vi "TestHB_Emb_1_arraysender.vi"() -> ()   [LabVIEW 2012]
doc: "SciScan 1.2 160622"
uses:
  SubVIs/Master Slave messaging Flags.ctl
  Custom Controls and Typedefs/HB_Error Conditions Cluster.ctl
  Custom Controls and Typedefs/Heartbeat information cluster.ctl
  Custom Controls and Typedefs/Heartbeat Event Source.ctl
  Custom Controls/Heartbeat_States.ctl
  SubVIs/Heartbeat state manager Input VI names.ctl
  Custom Controls and Typedefs/HB Actionable Event.ctl
  Custom Controls and Typedefs/HFG Commands.ctl
panel:
  in  "Cancel Sending":bool
  in  "Send command":bool
  out "Master instr received":i32
  out "Slave conf received":i32
  out "Heartbeat information cluster":T1
  out "Error conditions Cluster":T4
  out "Master-Slave messaging Flags":T5={"Instruction available"=TRUE, "Slave action completed"=TRUE, "Slave Ready?"=FALSE}
  in  "stop":bool
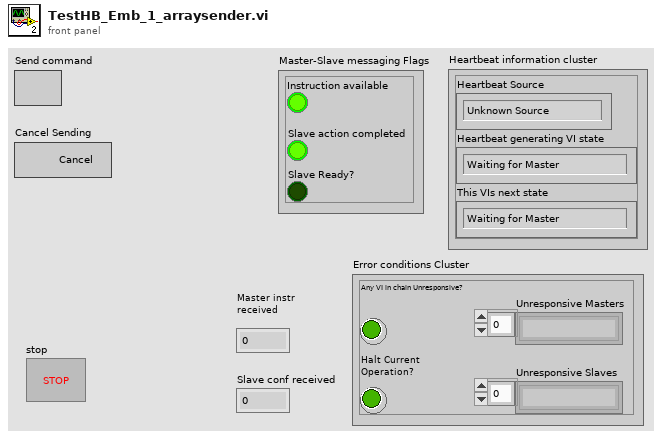
[diagram p1: front panel]
types:
  T1 = typedef "Heartbeat information cluster.ctl" = cluster{"Heartbeat Source":T2, "Heartbeat generating VI state":T3, "This VIs next state":T3}
  T2 = typedef "Heartbeat Event Source.ctl" = enum16{"Unknown Source", "Timeout", "This VI", "Master", "Slave"}
  T3 = typedef "Heartbeat_States.ctl" = enum16{"Waiting for Master", "Instruction Issued", "Waiting for Slave Completion", "Completed", "Cancelled", "Failed", "Broken Link"}
  T4 = typedef "HB_Error Conditions Cluster.ctl" = cluster{"Any VI in chain Unresponsive?":bool, "Halt Current Operation?":bool, "Unresponsive Masters":string[], "Unresponsive Slaves":string[]}
  T5 = typedef "Master Slave messaging Flags.ctl" = cluster{"Instruction available":bool, "Slave action completed":bool, "Slave Ready?":bool}
  T6 = enum8{"Enabled", "Disabled", "Disabled and Grayed Out"}
  T7 = typedef "HB Actionable Event.ctl" = enum16{"Master instruction event", "Slave ready event", "Slave unavailable event", "Cancelled or Failed event", "Slave action complete event", "QUIT", "Broken Link", "Recovered from Broken Link"}
  T8 = typedef "Heartbeat state manager Input VI names.ctl" = cluster{"Current VI name":string, "Master VI Names":string[], "Slave VI Names":string[]}
  T9 = typedef "HFG Commands.ctl" = enum16{"Set", "Get", "Initialize"}
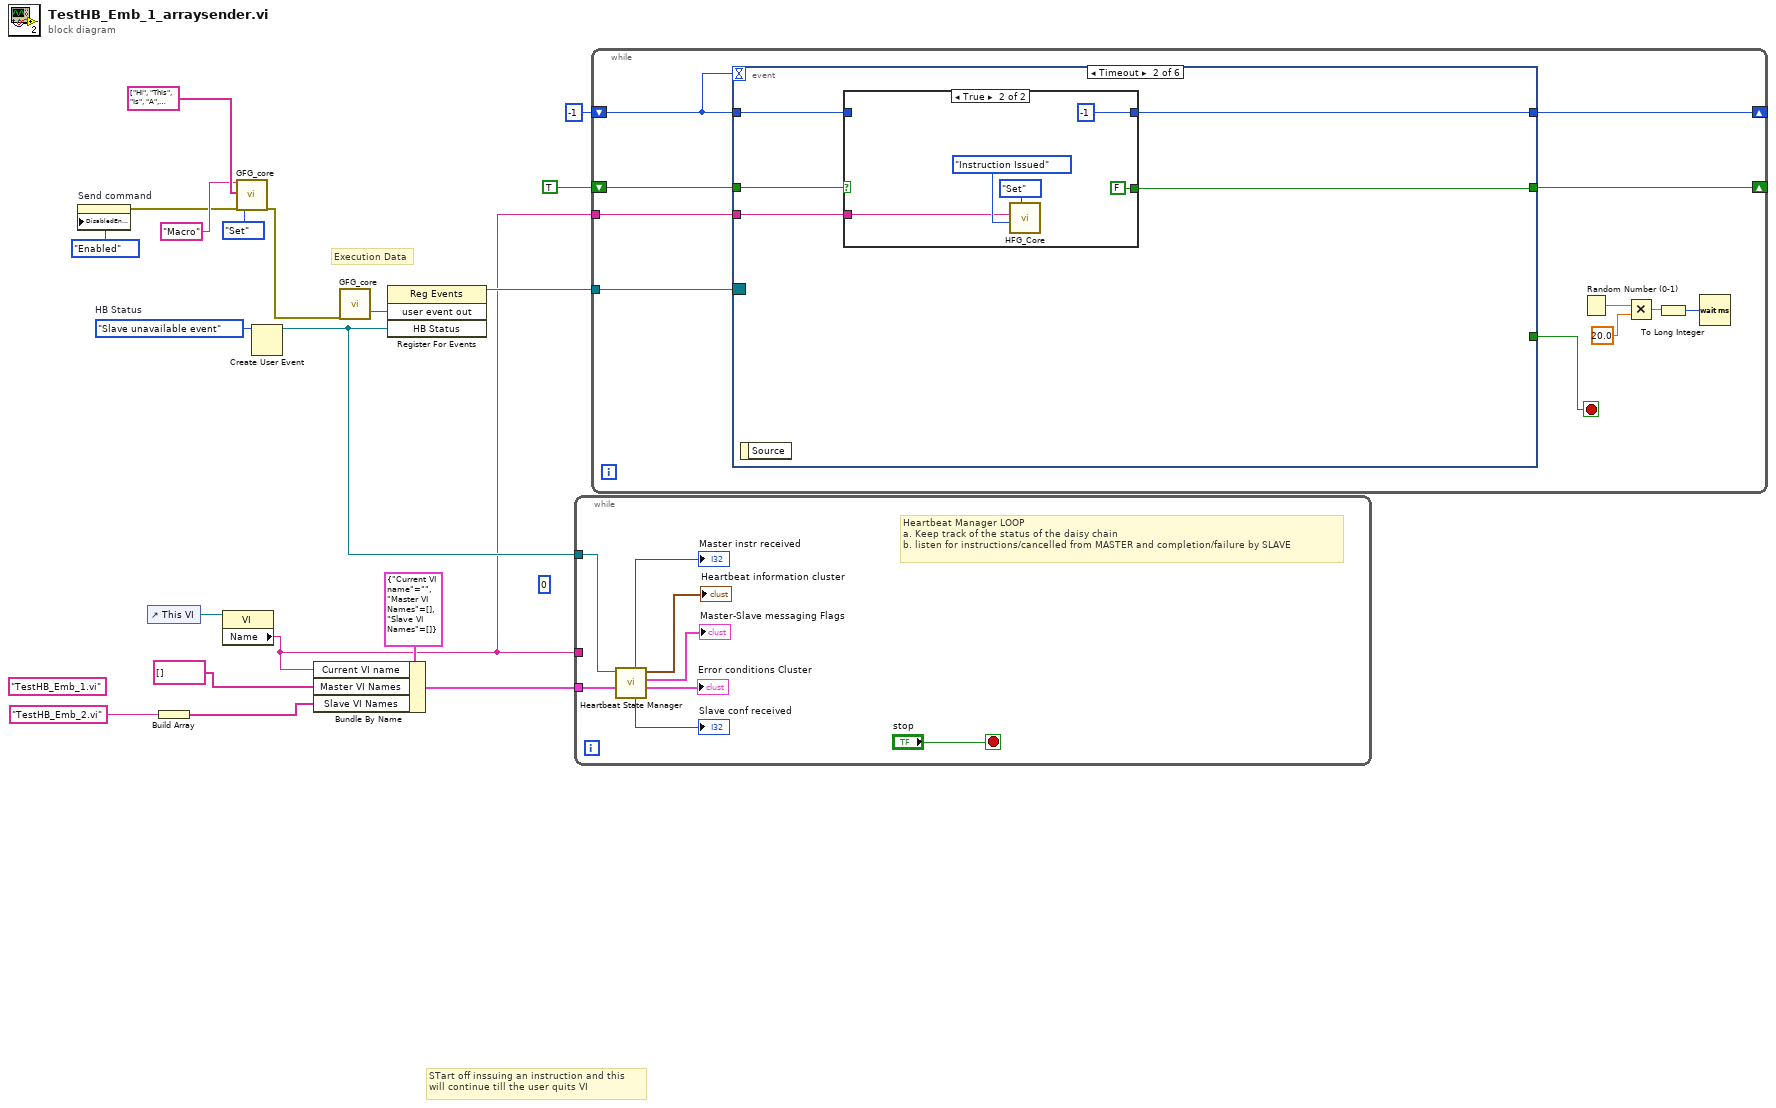
[diagram p0: block diagram]
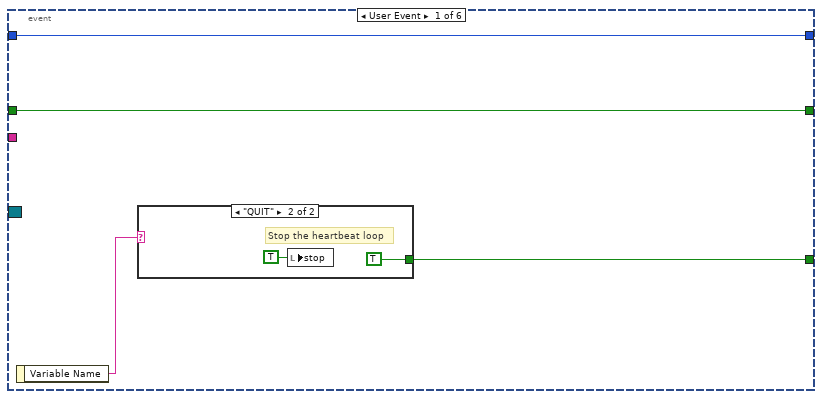
[diagram p2: hidden frame]
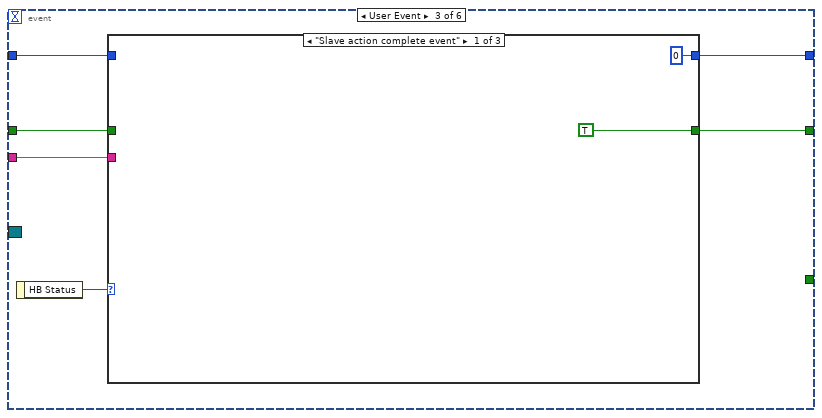
[diagram p5: hidden frame]
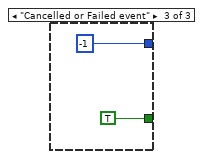
[diagram p7: hidden frame]
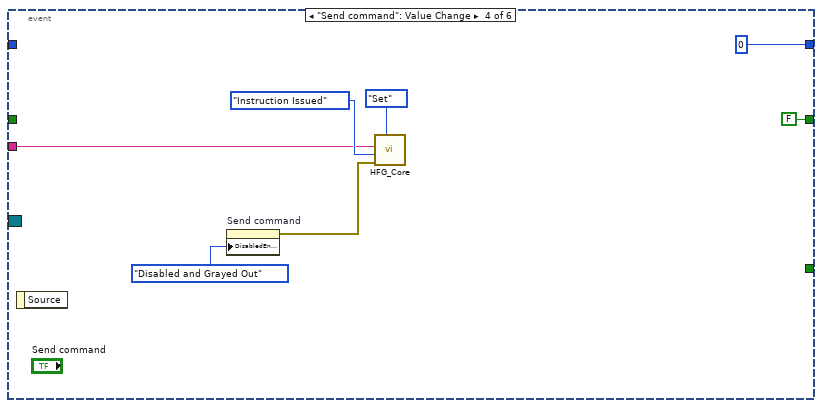
[diagram p8: hidden frame]
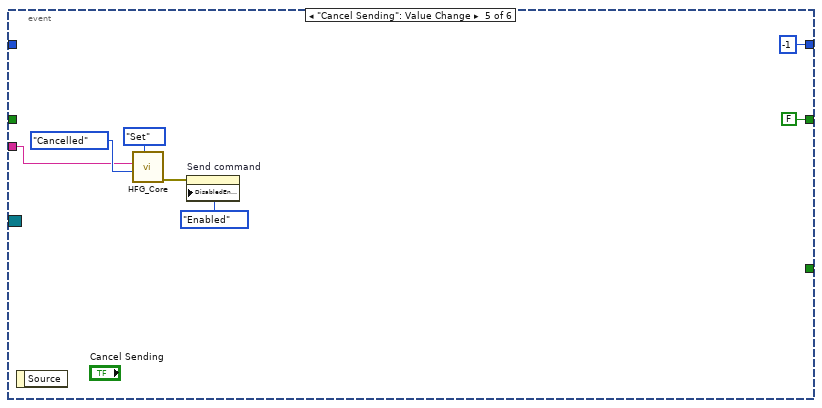
[diagram p9: hidden frame]
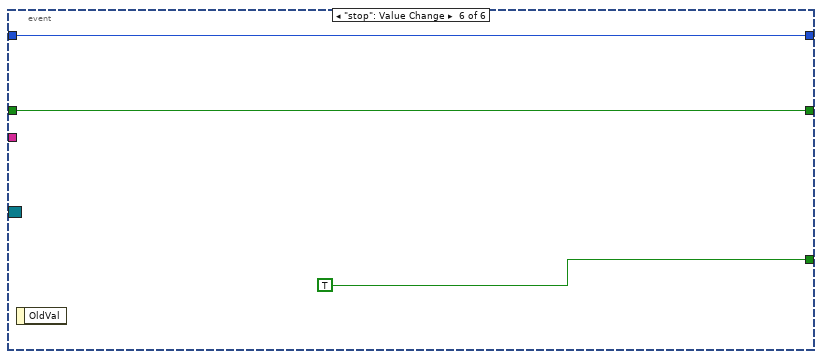
[diagram p10: hidden frame]
diagram:
  w12 = HB_Actionable_Event."Slave unavailable event"  # HB Status
  (unwired) 0
  (unwired) "TestHB_Emb_1.vi"
  # "STart off inssuing an instruction and this \nwill continue till the user quits VI"
  # "Execution Data"
  n1 = property on="Send command" class="Bool"("DisabledEnum"=T6."Enabled" ("Disabled")) -> (error out=w2:errorcluster)  [unwired: 2 in, 1 out]
  n2 = control-ref of="This VI"() -> (w17:refnum<vi>)
  n3 = Build Array("TestHB_Emb_2.vi") -> (w15:string[])
  n4 = property class="VI"(reference=w17) -> ("Name"=w9:string)  [unwired: 1 in, 2 out]
  n5 = call "GFG_core.vi"("Variable Name in"="Macro", "Variant in"=string[] ["Hi", "This", "Is", "A", "Test", "fg", "fgg", "ghg", "gh", "gh", "gh", "h", "hg", "f", "gn", "dghs", "dgh", "dghd", "dh", "d", "dghz", "afd", "gh", "afdg", "adfg", "dafg", "dfgh", "adfg", "dfg", "fdg", "dafg", "a", "hz", "fg", "dafg", "fdg", "adfg", "ag", "hadfg", "dfg", "adfg", "afg", "gjsgh", "dfhg", "dfg", "dfg", "jadfgh", "fhad", "hdgfh", "adfg", "hsdhgf", "adfg", "hdgfh", "fgg", "hdafh", "fdghfd", "hgsdha", "adfga", "ghadfh", "fdh", "fhjda", "fgasd", "hdha", "ahfdjhs", "dha", "hjg", "jgfsj", "adgh", "sdgh", "dsgjs", "adfh", "sdgha", "fdha", "dfhhs", "hgshjs", "gjhs", "gdh", "sgfh", "sgh", "gjhs", "hfdj", "dsfhj", "dfh", "jdhj", "fhjd", "ghfg", "fhjd", "dfjdf", "hjdf", "gjdfgj", "fhjd", "jkkg", "kfdh", "dfhjsd", "fhj", "fhj", "sfgj", "sfgjsf", "fgjgfj", "sfgjsf", "jfghjsgf", "fghjsf", "fsghj"] ("Array"), "error in (no error)"=w2, "Action"=enum16{"Init", "Set", "Get", "Clear"}."Set") -> ("error out"=w4:errorcluster)  [unwired: 9 in, 6 out]
  n6 = Create User Event(user event datatype=w12) -> (user event=w11:refnum<user-event>)  [unwired: 1 in, 1 out]
  n7 = Bundle By Name(cluster=T8 {"Current VI name"="", "Master VI Names"=[], "Slave VI Names"=[]} ("Heartbeat state manager Input VI names 2"), "Current VI name"=w9, "Master VI Names"=string[] [], "Slave VI Names"=w15) -> (w16:T8)
  n8 = call "GFG_core.vi"("error in (no error)"=w4) -> ("user event out"=w14:refnum<user-event>)  [unwired: 12 in, 6 out]
  n9 = register-events(w14, w11) -> (reference out=w13:refnum<event-registration>)  [unwired: 2 in, 1 out]
  n10 = while {
    tunnel: w16 -> [w27]
    tunnel: w9 -> [_]
    tunnel: w11 -> [w21]
    stop <- "stop" stop-if-true
    # "Heartbeat Manager LOOP \na. Keep track of the status of the daisy chain\nb. listen for instructions/cancelled from MASTER and completion/failure by SLAVE"
    n11 = call "Heartbeat State Manager.vi"("Heartbeat state manager Input VI names"=w27, "HB Command Event IN"=w21) -> ("Error conditions Cluster"=→"Error conditions Cluster":T4, "Master-Slave messaging Flags"=→"Master-Slave messaging Flags":T5, "Heartbeat information cluster"=→"Heartbeat information cluster":T1, "Slave Completions Received"=→"Slave conf received":i32, "Master Instructions Issued"=→"Master instr received":i32)  [unwired: 4 in, 1 out]
  }
  n12 = while {
    tunnel: w13 -> [w38]
    tunnel: w9 -> [w36]
    shift-right: [w34] -> _
    shift-left: TRUE ("slave ready") -> [w35]
    shift-right: [w29] -> _
    shift-left: -1 -> [w28]
    stop <- w37 stop-if-true
    n13 = event shown="[1] Timeout" {
      selector: w38 -> [_ _ _ _ _ _]
      dyn-events: _ -> [_ _ _ _ _ _]
      timeout: w28 -> [_ _ _ _ _ _]
      tunnel: [w41 _ _ _ _ TRUE] -> w37
      tunnel: w36 -> [_ w48 w61 w73 w80 _]
      tunnel: w35 -> [w40 w49 w60 _ _ w84]
      tunnel: [w40 w46 w59 FALSE ("slave ready") FALSE ("slave ready") w84] -> w34
      tunnel: [w39 w45 w57 0 -1 w83] -> w29
      tunnel: w28 -> [w39 w47 w58 _ _ w83]
      event User Event {
        n14 = event-data() -> ("Variable Name"=w42:string)  [unwired: 1 in]
        n15 = case shown="\"QUIT\"" w42 {
          tunnel: [_ TRUE] -> w41
          frame "False", Default {
          }
          frame "QUIT" {
            # "Stop the heartbeat loop"
            n16 = local write "stop"(TRUE ("stop")) -> ()
          }
        }
      }
      event Timeout {
        n17 = event-data() -> ()  [unwired: 1 in, 1 out]
        n18 = case shown="True" w49 {
          selector: w49 -> [w51 _]
          tunnel: w48 -> [_ w54]
          tunnel: w47 -> [w50 _]
          tunnel: [w51 FALSE] -> w46
          tunnel: [w50 -1] -> w45
          frame False {
          }
          frame True {
            n19 = call "HFG_Core.vi"("HFG Commands"=HFG_Commands."Set", "Heartbeat state IN"=Heartbeat_States."Instruction Issued", "VI Name (Calling VIs name by default)"=w54) -> ()  [unwired: 5 in, 4 out]
          }
        }
      }
      event User Event {
        n20 = event-data() -> ("HB Status"=w62:T7)  [unwired: 1 in]
        n21 = case shown="\"Slave action complete event\"" w62 {
          tunnel: w61 -> [_ _ _]
          tunnel: [TRUE ("slave ready") w66 TRUE ("slave ready")] -> w59
          tunnel: w60 -> [_ w66 _]
          tunnel: w58 -> [_ w65 _]
          tunnel: [0 w65 -1] -> w57
          frame "Slave action complete event" {
          }
          frame Default {
          }
          frame "Cancelled or Failed event" {
          }
        }
      }
      event "Send command": Value Change {
        n22 = event-data() -> ()  [unwired: 1 in, 1 out]
        n23 = property on="Send command" class="Bool"("DisabledEnum"=T6."Disabled and Grayed Out" ("Disabled")) -> (error out=w71:errorcluster)  [unwired: 2 in, 1 out]
        n24 = call "HFG_Core.vi"("HFG Commands"=HFG_Commands."Set", "Error In"=w71, "Heartbeat state IN"=Heartbeat_States."Instruction Issued", "VI Name (Calling VIs name by default)"=w73) -> ()  [unwired: 4 in, 4 out]
      }
      event "Cancel Sending": Value Change {
        n25 = event-data() -> ()  [unwired: 1 in, 1 out]
        n26 = call "HFG_Core.vi"("HFG Commands"=HFG_Commands."Set", "Heartbeat state IN"=Heartbeat_States."Cancelled", "VI Name (Calling VIs name by default)"=w80) -> ("Error Out"=w78:errorcluster)  [unwired: 5 in, 3 out]
        n27 = property on="Send command" class="Bool"(error in=w78, "DisabledEnum"=T6."Enabled" ("Disabled")) -> ()  [unwired: 1 in, 2 out]
      }
      event "stop": Value Change {
        n28 = event-data() -> ()  [unwired: 1 in, 1 out]
      }
    }
    n29 = Random Number (0-1)() -> (number: 0 to 1=w33:dbl)
    n30 = Multiply(x=w33, y=20.0) -> (x*y=w31:dbl)
    n31 = To Long Integer(number=w31) -> (32bit integer=w30:i32)
    n32 = Wait (ms)(milliseconds to wait=w30) -> ()  [unwired: 1 out]
  }
